vi "Transient--Const.vi"() -> (3 "Transient Command":string)   [LabVIEW 2017, in "Communications Library.lvlib"]
uses:
  Communications Library.lvlib
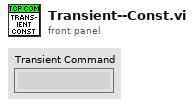
[diagram p1: front panel]
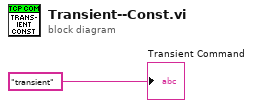
[diagram p0: block diagram]
diagram:
  "Transient Command" <- "transient" ("data in")
